vi "Create Dual Tone LUT.vi"(7 "output level units":T3, 11 "dual tone properties":T1) -> (3 "Signal Properties":T4)   [LabVIEW 2021, in "DigitalAudioGenerationProcess.lvlib"]
uses:
  DigitalAudioGenerationProcess.lvlib
  <vilib>/PDM Acquisition Toolkit/host/Classes/Tasks/I2S Output/Control/SignalProperties.ctl
  <vilib>/PDM Acquisition Toolkit/host/Classes/Channels/I2S Ouput/Controls/GenerationChannelProperties.ctl
  shared/controls/digital output level units.ctl
  controls/dual tone properties.ctl
  controls/dual tone types.ctl
  <vilib>/PDM Acquisition Toolkit/host/Classes/Channels/I2S Ouput/I2S Output Channel.lvclass
  <vilib>/PDM Acquisition Toolkit/host/Classes/Tasks/I2S Output/I2S Output Task.lvclass
  <vilib>/Analysis/NI_AALBase.lvlib
  <vilib>/gmath/NI_Gmath.lvlib
  shared/controls/audio controls.lvlib
  controls/AudioGenTypeDefs.lvlib
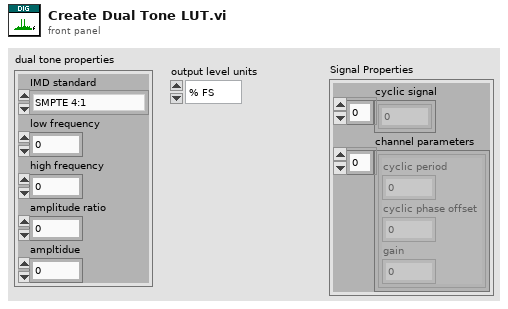
[diagram p1: front panel]
types:
  T1 = typedef "AudioGenTypeDefs.lvlib/dual tone properties.ctl" = cluster{"IMD standard":T2, "low frequency":dbl, "high frequency":dbl, "amplitude ratio":dbl, "ampltidue":dbl}
  T2 = typedef "AudioGenTypeDefs.lvlib/dual tone types.ctl" = enum32{"SMPTE 4:1", "DIN", "CCIF 11k-12k", "CCIF 19k-20k", "Custom"}
  T3 = typedef "audio controls.lvlib/digital output level units.ctl" = enum32{"% FS", "dBFS", "V"}
  T4 = typedef "PDM Acquisition Class Library.lvlib/I2S Output Task.lvclass/SignalProperties.ctl" = cluster{"cyclic signal":dbl[], "channel parameters":T5[]}
  T5 = typedef "PDM Acquisition Class Library.lvlib/I2S Output Channel.lvclass/GenerationChannelProperties.ctl" = cluster{"cyclic period":dbl, "cyclic phase offset":dbl, "gain":dbl}
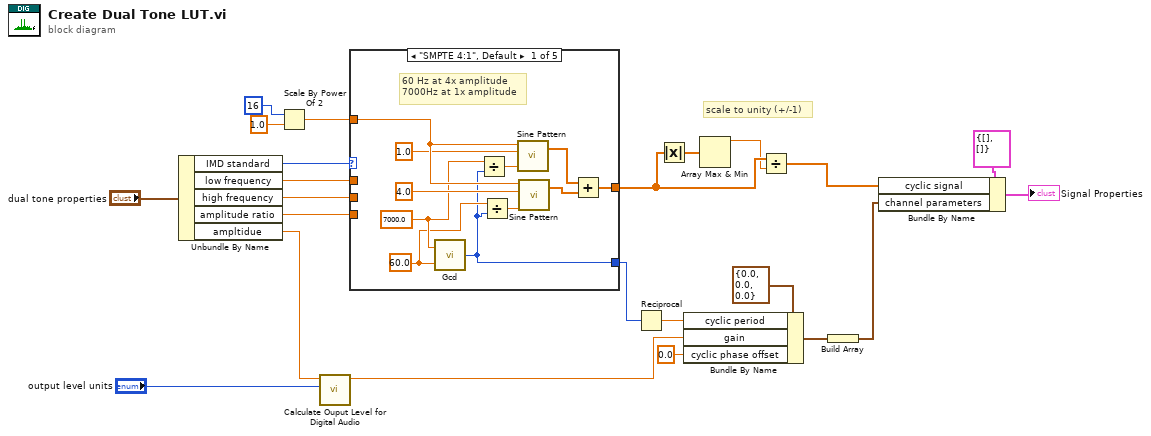
[diagram p0: block diagram]
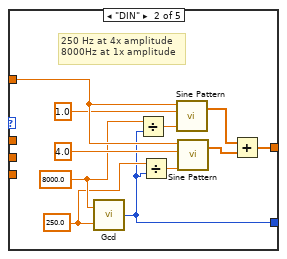
[diagram p2: hidden frame]
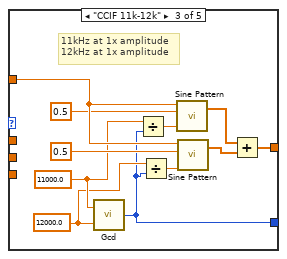
[diagram p3: hidden frame]
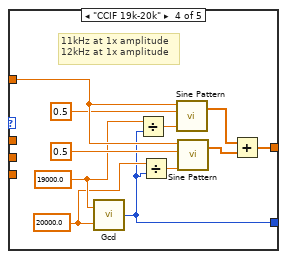
[diagram p4: hidden frame]
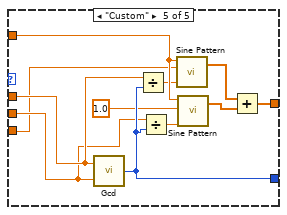
[diagram p5: hidden frame]
diagram:
  # "scale to unity (+/-1)"
  n1 = Unbundle By Name("dual tone properties") -> ("IMD standard"=w14:T2, "low frequency"=w13:dbl, "high frequency"=w12:dbl, "amplitude ratio"=w11:dbl, "ampltidue"=w15:dbl)
  n2 = Scale By Power Of 2(n=i16 16, x=1.0) -> (x*2^n=w8:dbl)
  n3 = call "Calculate Ouput Level for Digital Audio.vi"("digital output level units"="output level units", "output level"=w15) -> ("gain"=w18:dbl)  [unwired: 8 in, 1 out]
  n4 = case shown="\"SMPTE 4:1\", Default" w14 {
    tunnel: w13 -> [_ _ _ _ w71]
    tunnel: w12 -> [_ _ _ _ w70]
    tunnel: w11 -> [_ _ _ _ w69]
    tunnel: w8 -> [w32 w43 w54 w65 w76]
    tunnel: [w24 w35 w46 w57 w72] -> w7
    tunnel: [w31 w42 w53 w64 w75] -> w3
    frame "SMPTE 4:1", Default {
      w25 = 60.0 ("cycles")
      w27 = 7000.0 ("cycles")
      # "60 Hz at 4x amplitude\n7000Hz at 1x amplitude"
      n5 = call <vilib>:"Gcd.vi"("y"=w25, "x"=w27) -> ("gcd(x,y)"=w24:i32)
      n6 = Divide(x=w27, y=w24) -> (x/y=w28:dbl)
      n7 = Divide(x=w25, y=w24) -> (x/y=w26:dbl)
      n8 = call <vilib>:"Sine Pattern.vi"("cycles"=w28, "amplitude"=1.0, "samples"=w32) -> ("Sinusoidal Pattern"=w33:dbl[])  [unwired: 1 in, 1 out]
      n9 = call <vilib>:"Sine Pattern.vi"("cycles"=w26, "amplitude"=4.0, "samples"=w32) -> ("Sinusoidal Pattern"=w34:dbl[])  [unwired: 1 in, 1 out]
      n10 = Add(x=w33, y=w34) -> (x+y=w31:dbl[])
    }
    frame "DIN" {
      w36 = 250.0 ("cycles")
      w38 = 8000.0 ("cycles")
      # "250 Hz at 4x amplitude\n8000Hz at 1x amplitude"
      n11 = call <vilib>:"Gcd.vi"("y"=w36, "x"=w38) -> ("gcd(x,y)"=w35:i32)
      n12 = Divide(x=w38, y=w35) -> (x/y=w39:dbl)
      n13 = Divide(x=w36, y=w35) -> (x/y=w37:dbl)
      n14 = call <vilib>:"Sine Pattern.vi"("cycles"=w39, "amplitude"=1.0, "samples"=w43) -> ("Sinusoidal Pattern"=w44:dbl[])  [unwired: 1 in, 1 out]
      n15 = call <vilib>:"Sine Pattern.vi"("cycles"=w37, "amplitude"=4.0, "samples"=w43) -> ("Sinusoidal Pattern"=w45:dbl[])  [unwired: 1 in, 1 out]
      n16 = Add(x=w44, y=w45) -> (x+y=w42:dbl[])
    }
    frame "CCIF 11k-12k" {
      w47 = 12000.0 ("cycles")
      w49 = 11000.0 ("cycles")
      # "11kHz at 1x amplitude\n12kHz at 1x amplitude"
      n17 = call <vilib>:"Gcd.vi"("y"=w47, "x"=w49) -> ("gcd(x,y)"=w46:i32)
      n18 = Divide(x=w49, y=w46) -> (x/y=w50:dbl)
      n19 = Divide(x=w47, y=w46) -> (x/y=w48:dbl)
      n20 = call <vilib>:"Sine Pattern.vi"("cycles"=w50, "amplitude"=0.5, "samples"=w54) -> ("Sinusoidal Pattern"=w55:dbl[])  [unwired: 1 in, 1 out]
      n21 = call <vilib>:"Sine Pattern.vi"("cycles"=w48, "amplitude"=0.5, "samples"=w54) -> ("Sinusoidal Pattern"=w56:dbl[])  [unwired: 1 in, 1 out]
      n22 = Add(x=w55, y=w56) -> (x+y=w53:dbl[])
    }
    frame "CCIF 19k-20k" {
      w58 = 20000.0 ("cycles")
      w60 = 19000.0 ("cycles")
      # "11kHz at 1x amplitude\n12kHz at 1x amplitude"
      n23 = call <vilib>:"Gcd.vi"("y"=w58, "x"=w60) -> ("gcd(x,y)"=w57:i32)
      n24 = Divide(x=w60, y=w57) -> (x/y=w61:dbl)
      n25 = Divide(x=w58, y=w57) -> (x/y=w59:dbl)
      n26 = call <vilib>:"Sine Pattern.vi"("cycles"=w61, "amplitude"=0.5, "samples"=w65) -> ("Sinusoidal Pattern"=w66:dbl[])  [unwired: 1 in, 1 out]
      n27 = call <vilib>:"Sine Pattern.vi"("cycles"=w59, "amplitude"=0.5, "samples"=w65) -> ("Sinusoidal Pattern"=w67:dbl[])  [unwired: 1 in, 1 out]
      n28 = Add(x=w66, y=w67) -> (x+y=w64:dbl[])
    }
    frame "Custom" {
      n29 = call <vilib>:"Gcd.vi"("y"=w70, "x"=w71) -> ("gcd(x,y)"=w72:i32)
      n30 = Divide(x=w71, y=w72) -> (x/y=w74:dbl)
      n31 = Divide(x=w70, y=w72) -> (x/y=w73:dbl)
      n32 = call <vilib>:"Sine Pattern.vi"("cycles"=w74, "amplitude"=w69, "samples"=w76) -> ("Sinusoidal Pattern"=w77:dbl[])  [unwired: 1 in, 1 out]
      n33 = call <vilib>:"Sine Pattern.vi"("cycles"=w73, "amplitude"=1.0, "samples"=w76) -> ("Sinusoidal Pattern"=w78:dbl[])  [unwired: 1 in, 1 out]
      n34 = Add(x=w77, y=w78) -> (x+y=w75:dbl[])
    }
  }
  n35 = Reciprocal(x=w7) -> (1/x=w19:dbl)
  n36 = Absolute Value(x=w3) -> (abs(x)=w4:dbl[])
  n37 = Bundle By Name(cluster=T5 {"cyclic period"=0.0, "cyclic phase offset"=0.0, "gain"=0.0}, "cyclic period"=w19, "gain"=w18, "cyclic phase offset"=0.0) -> (w6:T5)
  n38 = Array Max & Min(array=w4) -> (max value=w2:dbl)  [unwired: 3 out]
  n39 = Divide(x=w3, y=w2) -> (x/y=w1:dbl[])
  n40 = Build Array(w6) -> (w5:T5[])
  n41 = Bundle By Name(cluster=T4 {"cyclic signal"=[], "channel parameters"=[]} ("Signal Properties"), "cyclic signal"=w1, "channel parameters"=w5) -> (→"Signal Properties":T4)
